vi "StageTest.vi"() -> ()   [LabVIEW 2020]
uses:
  PosCtrlOptions.ctl
  SettingCtrlOptions.ctl
panel:
  in  "Correction Table Path":path
  in  "Speed":sgl
  in  "Move to":sgl[](array[numeric])
  out "XY Graph":cluster{sgl[], sgl[]}(graph)
  out "Position":sgl[](array[numeric])
  in  "Stop":bool
  in  "Step Sizes(mm)":dbl[](array[numeric])
  out "IDs":i32[](array[numeric])
  out "Serial nos":u32[](array[numeric])
  out "Num of Controllers":i32
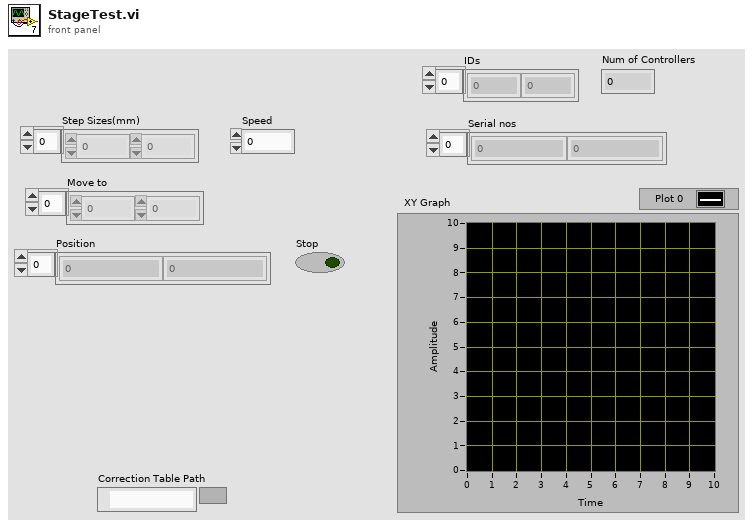
[diagram p1: front panel]
types:
  T1 = typedef "SettingCtrlOptions.ctl" = enum16{"Set X", "Set Y", "Set X and Y", "Get Settings", "None"}
  T2 = typedef "PosCtrlOptions.ctl" = enum16{"Move X", "Move Y", "Both X and Y", "Read Pos", "None"}
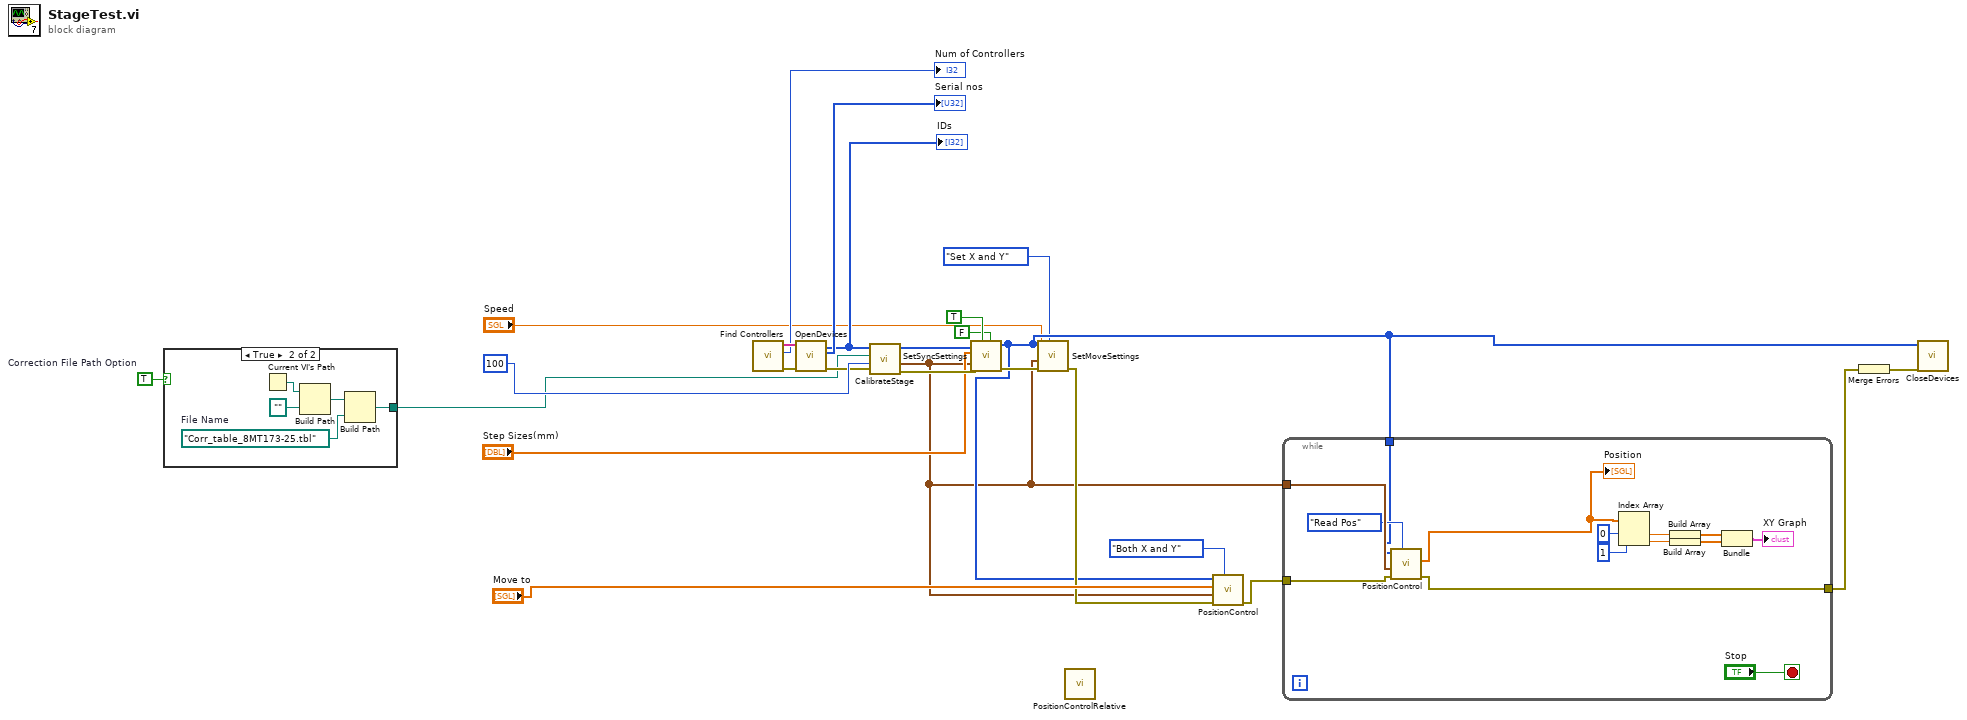
[diagram p0: block diagram]
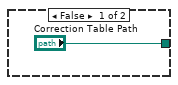
[diagram p2: hidden frame]
diagram:
  w2 = TRUE  # Correction File Path Option
  n1 = case shown="True" w2 {
    tunnel: ["Correction Table Path" w27] -> w1
    frame False {
    }
    frame True {
      w28 = path "Corr_table_8MT173-25.tbl"  # File Name
      n2 = Current VI's Path() -> (path=w30:path)
      n3 = Build Path(base path=w30, name or relative path=path "") -> (appended path=w29:path)
      n4 = Build Path(base path=w29, name or relative path=w28) -> (appended path=w27:path)
    }
  }
  n5 = call "Find Controllers.vi"() -> ("error out"=w24:errorcluster, "Num of Controllers"=→"Num of Controllers":i32, "Names"=w25:string[])  [unwired: 9 in]
  n6 = call "OpenDevices.vi"("error In"=w24, "Names"=w25) -> ("error out"=w17:errorcluster, "Serial nos"=→"Serial nos":u32[], "IDs"=w15:i32[])  [unwired: 6 in]
  "IDs" <- w15
  n7 = call "CalibrateStage.vi"("error in (no error)"=w17, "numSteps = 1mm"=100, "Correction Table Path"=w1, "IDs"=w15) -> ("error out"=w16:errorcluster, "Calibration"=w4:cluster{dbl, "MicrostepMode":u32}[], "IDs Out"=w19:i32[])  [unwired: 2 in, 3 out]
  n8 = call "SetSyncSettings.vi"("Y SyncOut Enabled"=FALSE, "X SyncOut Enabled"=TRUE, "error in (no error)"=w16, "Calibration"=w4, "Step Sizes(mm)"="Step Sizes(mm)", "IDs"=w19) -> ("error out"=w7:errorcluster, "IDs Out"=w6:i32[])  [unwired: 4 in]
  n9 = call "SetMoveSettings.vi"("Mode"=SettingCtrlOptions."Set X and Y", "error in (no error)"=w7, "Calibration"=w4, "Speed"="Speed", "IDs"=w6) -> ("error out"=w8:errorcluster)  [unwired: 4 in, 2 out]
  n10 = call "PositionControlRelative.vi"() -> ()  [unwired: 9 in, 3 out]
  n11 = call "PositionControl.vi"("Mode"=PosCtrlOptions."Both X and Y", "error in (no error)"=w8, "Calibration"=w4, "Move to"="Move to", "IDs"=w6) -> ("error out"=w9:errorcluster)  [unwired: 4 in, 2 out]
  n12 = while {
    tunnel: w6 -> [w34]
    tunnel: [w32] -> w12
    tunnel: w9 -> [w37]
    tunnel: w4 -> [w36]
    stop <- "Stop" stop-if-true
    n13 = call "PositionControl.vi"("Mode"=PosCtrlOptions."Read Pos", "error in (no error)"=w37, "Calibration"=w36, "IDs"=w34) -> ("error out"=w32:errorcluster, "Position"=w33:sgl[])  [unwired: 5 in, 1 out]
    "Position" <- w33
    n14 = Index Array(array=w33, index #1=0 ("index"), index #2=1 ("index")) -> (element #1=w41:sgl, element #2=w42:sgl)
    n15 = Build Array(w41) -> (w39:sgl[])
    n16 = Build Array(w42) -> (w38:sgl[])
    n17 = Bundle(w39, w38) -> (→"XY Graph":cluster{sgl[], sgl[]})  [unwired: 1 in]
  }
  n18 = Merge Errors(w12) -> (w13:errorcluster)
  n19 = call "CloseDevices.vi"("error in (no error)"=w13, "Ids"=w6) -> ()  [unwired: 9 in, 1 out]
